vi "test.vi"() -> ()   [LabVIEW 2010, in "XMLElement.lvclass"]
uses:
  XMLElement.lvclass
panel:
  in  "treat as XML":bool
  in  "root tag":string="root"
  in  "ignore IDs (just find first element)?":bool
  in  "attribute (setting)":string caption="attribute"
  in  "content (setting)":string caption="content"
  in  "set element at":bool
  in  "id chain (setting)":string[](array[string]) caption="id chain"
  in  "name chain (setting)":string[](array[string]) caption="name chain"
  in  "attribute (fetching)":string caption="attribute"
  out "content (fetching)":string caption="content"
  in  "fetch content at":bool
  in  "id chain (fetching)":string[](array[string]) caption="id chain"
  in  "name chain (fetching)":string[](array[string]) caption="name chain"
  in  "ID attribute name (for building)":string="ID" caption="ID attribute name"
  in  "ID attribute name (for parsing)":string="ID" caption="ID attribute name"
  in  "parse button":bool
  in  "XML input":string
  out "XML string":string
  in  "stop":bool
  # "Test program for Element.lvclass"
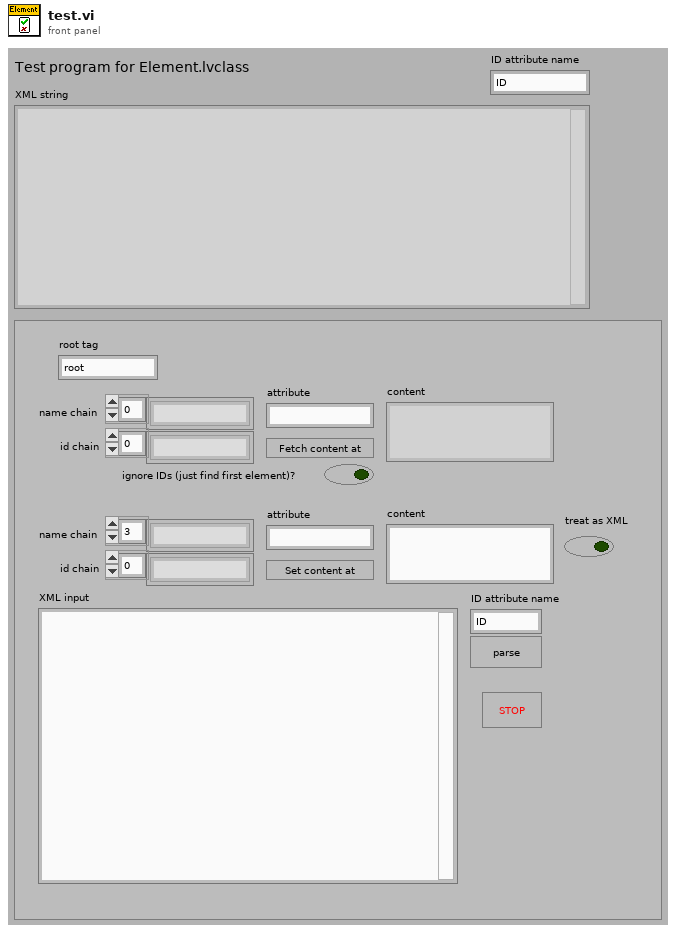
[diagram p1: front panel]
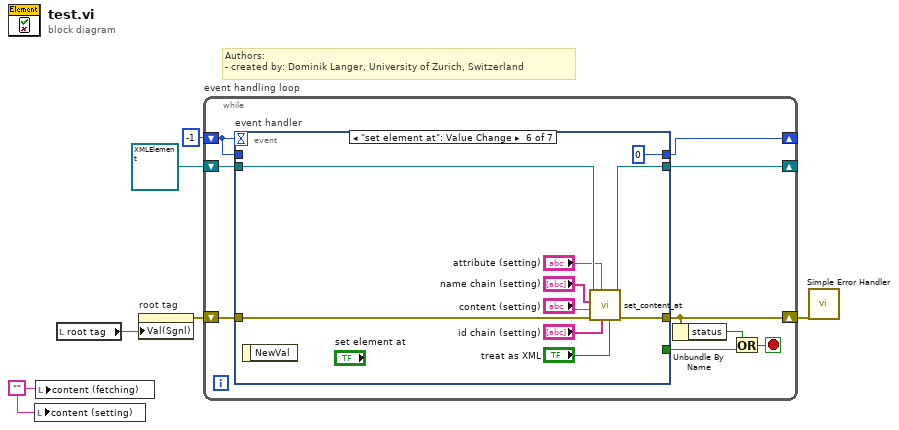
[diagram p0: block diagram]
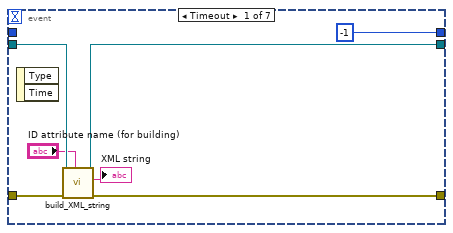
[diagram p2: hidden frame]
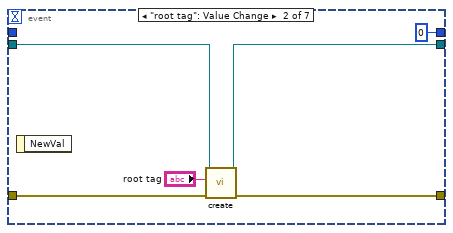
[diagram p3: hidden frame]
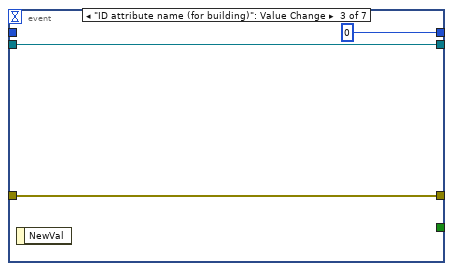
[diagram p4: hidden frame]
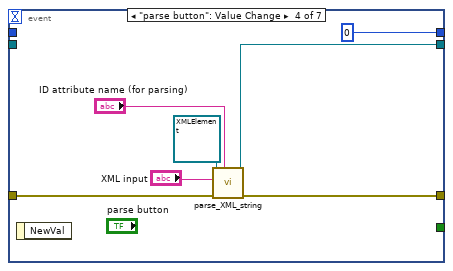
[diagram p5: hidden frame]
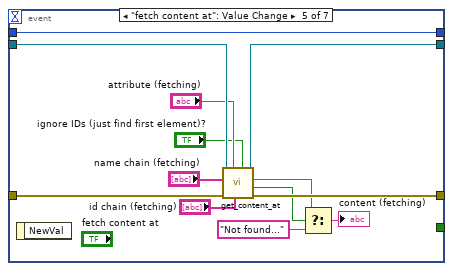
[diagram p6: hidden frame]
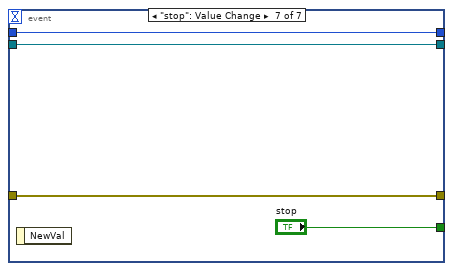
[diagram p7: hidden frame]
diagram:
  w4 = ""
  # "Authors: \n- created by: Dominik Langer, University of Zurich, Switzerland"
  n1 = local write "content (setting)"(w4) -> ()
  n2 = local write "content (fetching)"(w4) -> ()
  n3 = local read "root tag"() -> (w2:string)
  n4 = property on="root tag" class="Str"("Val(Sgnl)"=w2) -> (error out=w1:errorcluster)  [unwired: 2 in, 1 out]
  n5 = while "event handling loop" {
    shift-right: [w12] -> _
    shift-left: refnum<class "XMLElement.lvclass"> refnum ("Element.lvclass") -> [w15]
    shift-right: [w11] -> _
    shift-left: -1 -> [w14]
    shift-right: [w10] -> w3
    shift-left: w1 -> [w13]
    stop <- w7 stop-if-true
    n6 = event "event handler" shown="[5] \"set element at\": Value Change" {
      selector: _ -> [_ _ _ _ _ _ _]
      dyn-events: _ -> [_ _ _ _ _ _ _]
      timeout: w14 -> [_ _ _ _ _ _ _]
      tunnel: w15 -> [w19 w26 w30 _ w47 w59 w64]
      tunnel: w14 -> [_ _ _ _ w51 _ w62]
      tunnel: w13 -> [w20 w28 w31 w38 w48 w61 w65]
      tunnel: [w16 w27 w31 w37 w46 w60 w65] -> w10
      tunnel: [w17 w25 w30 w36 w45 w58 w64] -> w12
      tunnel: [_ _ _ _ _ _ "stop"] -> w8
      tunnel: [-1 0 0 0 w51 0 w62] -> w11
      event Timeout {
        n7 = event-data() -> ()  [unwired: 1 in, 2 out]
        n8 = call "build_XML_string.vi"("ID tag"="ID attribute name (for building)", "error in (no error)"=w20, "Element in"=w19) -> ("error out"=w16:errorcluster, "string"=→"XML string":string, "Element out"=w17:refnum<class "XMLElement.lvclass">)  [unwired: 6 in]
      }
      event "root tag": Value Change {
        n9 = event-data() -> ()  [unwired: 1 in, 1 out]
        n10 = call "create.vi"("error in (no error)"=w28, "name"="root tag", "XMLElement in"=w26) -> ("error out"=w27:errorcluster, "XMLElement out"=w25:refnum<class "XMLElement.lvclass">)  [unwired: 7 in]
      }
      event "ID attribute name (for building)": Value Change {
        n11 = event-data() -> ()  [unwired: 1 in, 1 out]
      }
      event "parse button": Value Change {
        n12 = event-data() -> ()  [unwired: 1 in, 1 out]
        n13 = call "parse_XML_string.vi"("ID attribute"="ID attribute name (for parsing)", "error in (no error)"=w38, "XML string"="XML input", "Element in"=refnum<class "XMLElement.lvclass"> refnum ("Element.lvclass")) -> ("error out"=w37:errorcluster, "Element out"=w36:refnum<class "XMLElement.lvclass">)  [unwired: 6 in]
      }
      event "fetch content at": Value Change {
        n14 = event-data() -> ()  [unwired: 1 in, 1 out]
        n15 = call "get_content_at.vi"("ignore IDs"="ignore IDs (just find first element)?", "ID chain"="id chain (fetching)", "attribute name"="attribute (fetching)", "error in (no error)"=w48, "key chain"="name chain (fetching)", "Element in"=w47) -> ("error out"=w46:errorcluster, "found?"=w42:bool, "string"=w43:string, "Element out"=w45:refnum<class "XMLElement.lvclass">)  [unwired: 2 in]
        n16 = Select(t=w43, s=w42, f="Not found...") -> (s? t:f=→"content (fetching)":string)
      }
      event "set element at": Value Change {
        n17 = event-data() -> ()  [unwired: 1 in, 1 out]
        n18 = call "set_content_at.vi"("value is XML itself?"="treat as XML", "id chain"="id chain (setting)", "attribute name"="attribute (setting)", "error in (no error)"=w61, "content"="content (setting)", "key chain"="name chain (setting)", "Element in"=w59) -> ("error out"=w60:errorcluster, "Element out"=w58:refnum<class "XMLElement.lvclass">)  [unwired: 3 in]
      }
      event "stop": Value Change {
        n19 = event-data() -> ()  [unwired: 1 in, 1 out]
      }
    }
    n20 = Unbundle By Name(w10) -> ("status"=w9:bool)
    n21 = Or(x=w9, y=w8) -> (x .or. y?=w7:bool)
  }
  n22 = call <vilib>:"Simple Error Handler.vi"("error in (no error)"=w3) -> ()  [unwired: 4 in, 5 out]
